vi "Window In Front.vi"   [LabVIEW 2014]
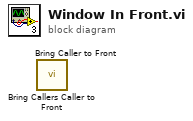
[diagram p0: block diagram]
diagram:
  n1 = call "Bring Callers Caller to Front.vi"() -> ()  [unwired: 11 in, 1 out]
  n2 = call "Bring Caller to Front.vi"() -> ()  [unwired: 11 in, 1 out]
